vi "Least squares solution.vi"(0 "Y":T1 caption="Y（误差）", 5 "PWM数组":dbl[](array[numeric])) -> (2 "PWM8":dbl, 3 "PWM6":dbl, 4 "PWM1":dbl, 6 "PWM2":dbl, 8 "PWM3":dbl, 10 "PWM4":dbl, 13 "PWM9":dbl, 14 "PWM7":dbl, 15 "PWM5":dbl)   [LabVIEW 2017]
uses:
  <vilib>/Analysis/Matrix/Datatypes/RealMatrix.ctl
  <vilib>/Analysis/_algsub.llb/Real Matrix Condition Number.vi
  <vilib>/Analysis/baseanly.llb/Real A x B.vi
  <vilib>/Analysis/Matrix/Numeric/Add/Add - RM,RM.vi
  <vilib>/Analysis/baseanly.llb/Real Inverse Matrix.vi
  <vilib>/Analysis/NI_AALBase.lvlib
  <vilib>/Analysis/NI_AALPro.lvlib
  <vilib>/Analysis/Matrix/NI_Matrix.lvlib
panel:
  out "condition number 2":dbl caption="条件数" format="%.4f"
  out "x*y":dbl[][](array[numeric])
  out "A + B":T1
  out "condition number":dbl caption="条件数" format="%.4f"
  out "Inverse Matrix":T1 caption="逆矩阵"
  out "矩阵A x B":T1
  out "S表":dbl[][](array[numeric])
  out "X":T1 caption="X（pwm/灯塔pwm）"
  # "横坐标是灯板编号\n纵坐标是传感器编号"
  # "PWM的变化量"
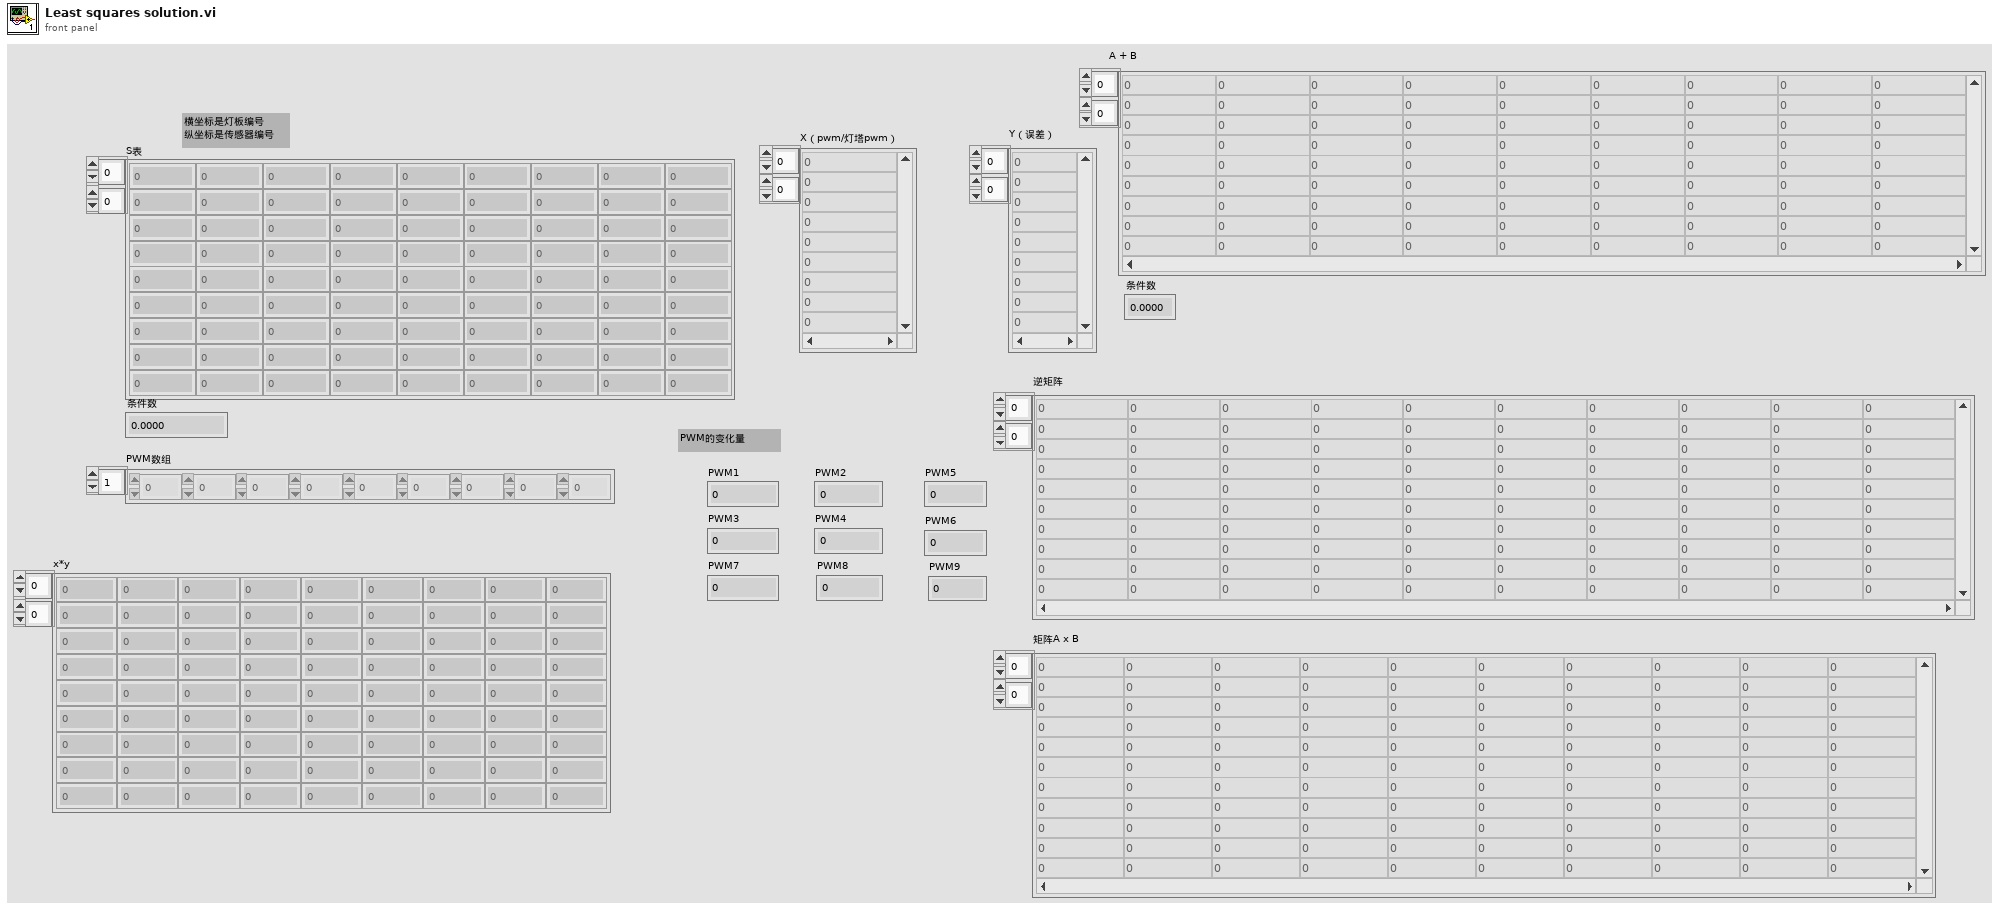
[diagram p1: front panel]
types:
  T1 = typedef "NI_Matrix.lvlib/RealMatrix.ctl" = dbl[][]
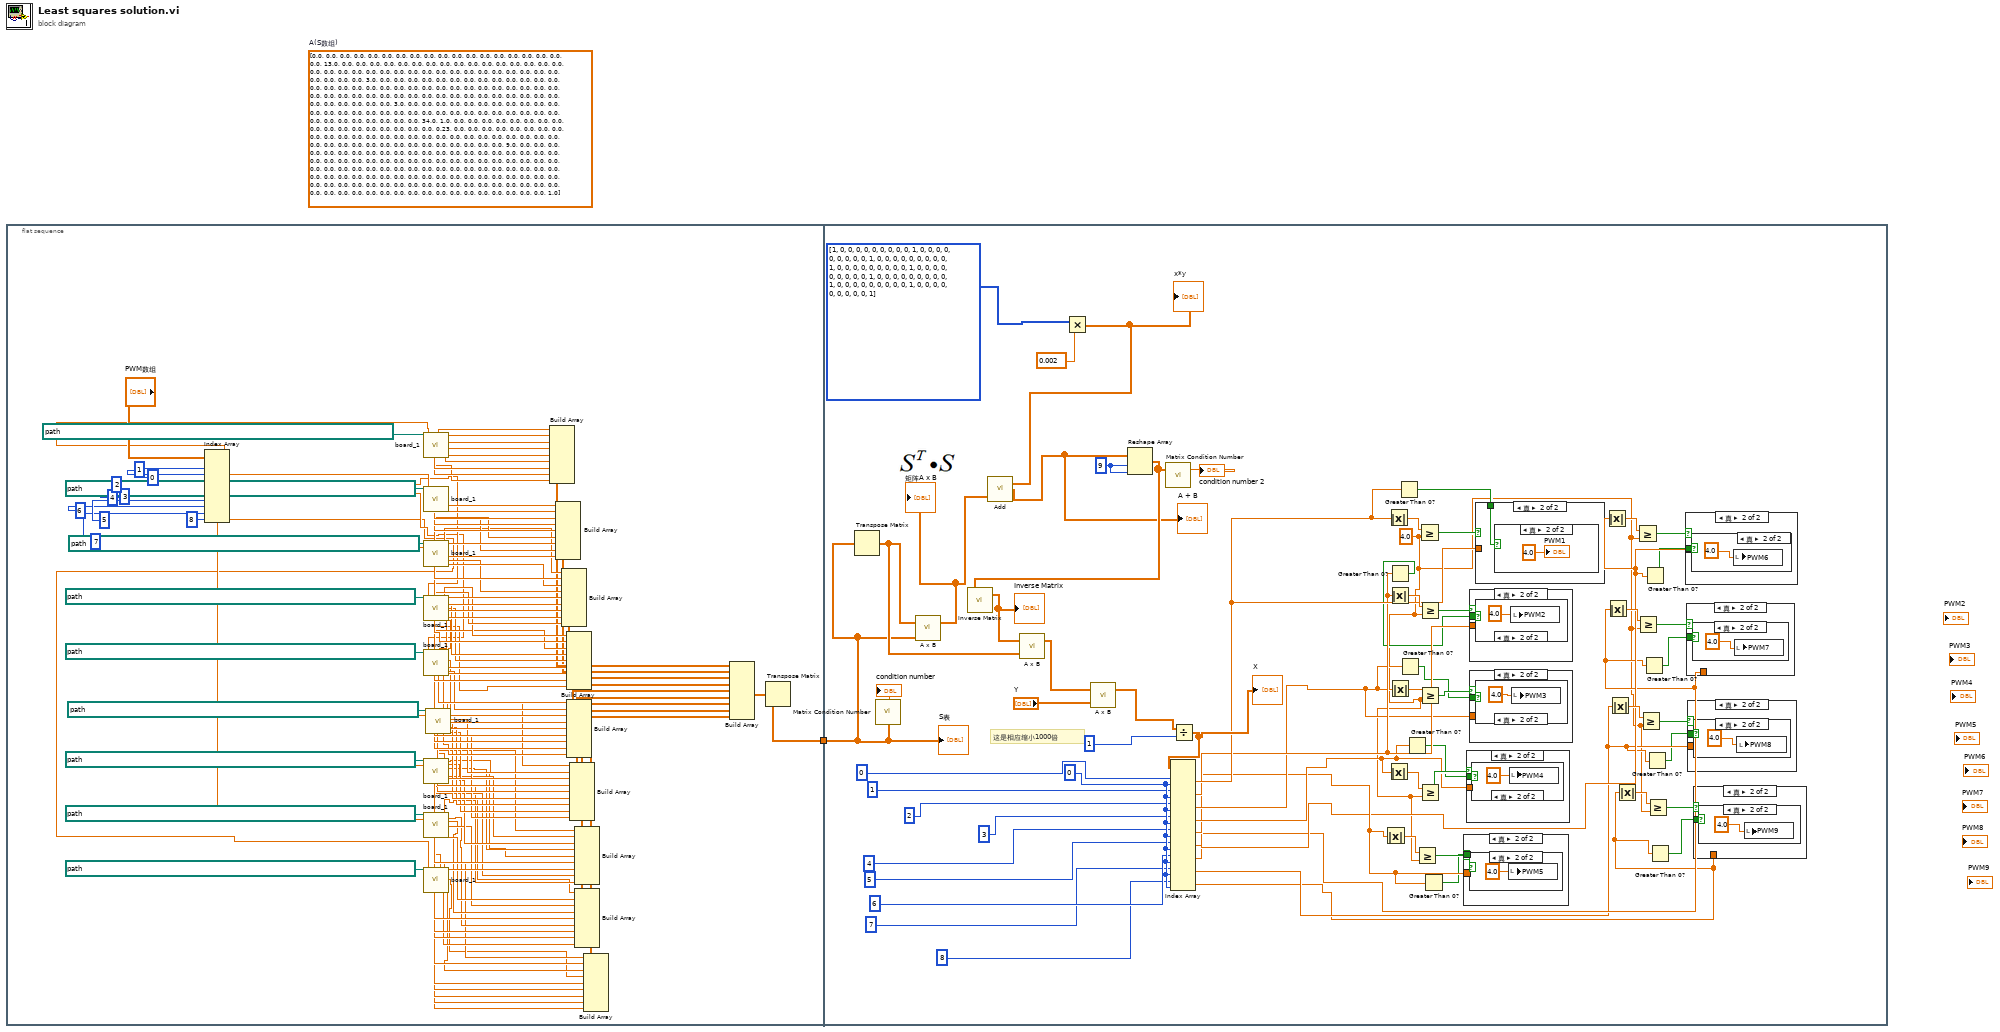
[diagram p0: block diagram]
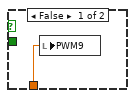
[diagram p2: hidden frame]
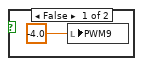
[diagram p3: hidden frame]
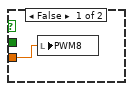
[diagram p4: hidden frame]
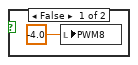
[diagram p5: hidden frame]
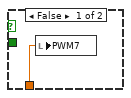
[diagram p6: hidden frame]
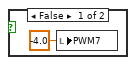
[diagram p7: hidden frame]
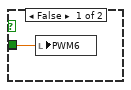
[diagram p8: hidden frame]
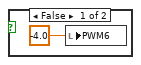
[diagram p9: hidden frame]
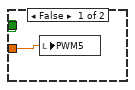
[diagram p10: hidden frame]
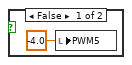
[diagram p11: hidden frame]
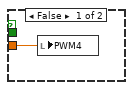
[diagram p12: hidden frame]
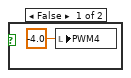
[diagram p13: hidden frame]
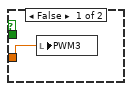
[diagram p14: hidden frame]
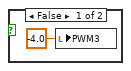
[diagram p15: hidden frame]
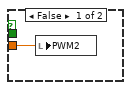
[diagram p16: hidden frame]
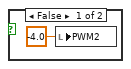
[diagram p17: hidden frame]
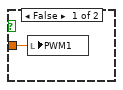
[diagram p18: hidden frame]
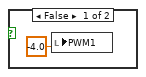
[diagram p19: hidden frame]
diagram:
  (unwired) dbl[][] [[0.0, 0.0, 0.0, 0.0, 0.0, 0.0, 0.0, 0.0, 0.0, 0.0, 0.0, 0.0, 0.0, 0.0, 0.0, 0.0, 0.0, 0.0], [0.0, 13.0, 0.0, 0.0, 0.0, 0.0, 0.0, 0.0, 0.0, 0.0, 0.0, 0.0, 0.0, 0.0, 0.0, 0.0, 0.0, 0.0], [0.0, 0.0, 0.0, 0.0, 0.0, 0.0, 0.0, 0.0, 0.0, 0.0, 0.0, 0.0, 0.0, 0.0, 0.0, 0.0, 0.0, 0.0], [0.0, 0.0, 0.0, 0.0, 3.0, 0.0, 0.0, 0.0, 0.0, 0.0, 0.0, 0.0, 0.0, 0.0, 0.0, 0.0, 0.0, 0.0], [0.0, 0.0, 0.0, 0.0, 0.0, 0.0, 0.0, 0.0, 0.0, 0.0, 0.0, 0.0, 0.0, 0.0, 0.0, 0.0, 0.0, 0.0], [0.0, 0.0, 0.0, 0.0, 0.0, 0.0, 0.0, 0.0, 0.0, 0.0, 0.0, 0.0, 0.0, 0.0, 0.0, 0.0, 0.0, 0.0], [0.0, 0.0, 0.0, 0.0, 0.0, 0.0, 3.0, 0.0, 0.0, 0.0, 0.0, 0.0, 0.0, 0.0, 0.0, 0.0, 0.0, 0.0], [0.0, 0.0, 0.0, 0.0, 0.0, 0.0, 0.0, 0.0, 0.0, 0.0, 0.0, 0.0, 0.0, 0.0, 0.0, 0.0, 0.0, 0.0], [0.0, 0.0, 0.0, 0.0, 0.0, 0.0, 0.0, 0.0, 34.0, 1.0, 0.0, 0.0, 0.0, 0.0, 0.0, 0.0, 0.0, 0.0], [0.0, 0.0, 0.0, 0.0, 0.0, 0.0, 0.0, 0.0, 0.0, 0.23, 0.0, 0.0, 0.0, 0.0, 0.0, 0.0, 0.0, 0.0], [0.0, 0.0, 0.0, 0.0, 0.0, 0.0, 0.0, 0.0, 0.0, 0.0, 0.0, 0.0, 0.0, 0.0, 0.0, 0.0, 0.0, 0.0], [0.0, 0.0, 0.0, 0.0, 0.0, 0.0, 0.0, 0.0, 0.0, 0.0, 0.0, 0.0, 0.0, 0.0, 9.0, 0.0, 0.0, 0.0], [0.0, 0.0, 0.0, 0.0, 0.0, 0.0, 0.0, 0.0, 0.0, 0.0, 0.0, 0.0, 0.0, 0.0, 0.0, 0.0, 0.0, 0.0], [0.0, 0.0, 0.0, 0.0, 0.0, 0.0, 0.0, 0.0, 0.0, 0.0, 0.0, 0.0, 0.0, 0.0, 0.0, 0.0, 0.0, 0.0], [0.0, 0.0, 0.0, 0.0, 0.0, 0.0, 0.0, 0.0, 0.0, 0.0, 0.0, 0.0, 0.0, 0.0, 0.0, 0.0, 0.0, 0.0], [0.0, 0.0, 0.0, 0.0, 0.0, 0.0, 0.0, 0.0, 0.0, 0.0, 0.0, 0.0, 0.0, 0.0, 0.0, 0.0, 0.0, 0.0], [0.0, 0.0, 0.0, 0.0, 0.0, 0.0, 0.0, 0.0, 0.0, 0.0, 0.0, 0.0, 0.0, 0.0, 0.0, 0.0, 0.0, 0.0], [0.0, 0.0, 0.0, 0.0, 0.0, 0.0, 0.0, 0.0, 0.0, 0.0, 0.0, 0.0, 0.0, 0.0, 0.0, 0.0, 0.0, 1.0]]  # A(S数组)
  n1 = flat-sequence {
    tunnel: [w11] -> w1
    tunnel: w1 -> [w125]
    frame #0 {
      n2 = Index Array(array="PWM数组", index #1=0 ("索引"), index #2=1 ("索引"), index #3=2 ("索引"), index #4=3 ("索引"), index #5=4 ("索引"), index #6=5 ("索引"), index #7=6 ("索引"), index #8=7 ("索引"), index #9=8 ("索引")) -> (element #1=w111:dbl, element #2=w19:dbl, element #3=w18:dbl, element #4=w17:dbl, element #5=w16:dbl, element #6=w15:dbl, element #7=w14:dbl, element #8=w13:dbl, element #9=w12:dbl)
      n3 = call "board_1.vi"("文件（使用对话框）"=path "D:/桌面文件/自动备份/自动匀光/程序/labview36/raw_data/S_rawdata_b1.txt", "PWM1"=w111) -> ("S1"=w110:dbl, "S2"=w109:dbl, "S3"=w108:dbl, "S4"=w107:dbl, "S5"=w106:dbl, "S6"=w105:dbl, "S7"=w104:dbl, "S8"=w103:dbl, "S9"=w102:dbl)  [unwired: 17 in]
      n4 = call "board_1.vi"("文件（使用对话框）"=path "D:/桌面文件/自动备份/自动匀光/程序/labview36/raw_data/S_rawdata_b2.txt", "PWM1"=w19) -> ("S1"=w101:dbl, "S2"=w100:dbl, "S3"=w99:dbl, "S4"=w98:dbl, "S5"=w97:dbl, "S6"=w96:dbl, "S7"=w95:dbl, "S8"=w94:dbl, "S9"=w93:dbl)  [unwired: 17 in]
      n5 = call "board_1.vi"("文件（使用对话框）"=path "D:/桌面文件/自动备份/自动匀光/程序/labview36/raw_data/S_rawdata_b3.txt", "PWM1"=w18) -> ("S1"=w92:dbl, "S2"=w91:dbl, "S3"=w90:dbl, "S4"=w89:dbl, "S5"=w88:dbl, "S6"=w87:dbl, "S7"=w86:dbl, "S8"=w85:dbl, "S9"=w84:dbl)  [unwired: 17 in]
      n6 = call "board_1.vi"("文件（使用对话框）"=path "D:/桌面文件/自动备份/自动匀光/程序/labview36/raw_data/S_rawdata_b4.txt", "PWM1"=w17) -> ("S1"=w83:dbl, "S2"=w82:dbl, "S3"=w81:dbl, "S4"=w80:dbl, "S5"=w79:dbl, "S6"=w78:dbl, "S7"=w77:dbl, "S8"=w76:dbl, "S9"=w75:dbl)  [unwired: 17 in]
      n7 = call "board_1.vi"("文件（使用对话框）"=path "D:/桌面文件/自动备份/自动匀光/程序/labview36/raw_data/S_rawdata_b5.txt", "PWM1"=w16) -> ("S1"=w74:dbl, "S2"=w73:dbl, "S3"=w72:dbl, "S4"=w71:dbl, "S5"=w70:dbl, "S6"=w69:dbl, "S7"=w68:dbl, "S8"=w67:dbl, "S9"=w66:dbl)  [unwired: 17 in]
      n8 = call "board_1.vi"("文件（使用对话框）"=path "D:/桌面文件/自动备份/自动匀光/程序/labview36/raw_data/S_rawdata_b7.txt", "PWM1"=w14) -> ("S1"=w56:dbl, "S2"=w55:dbl, "S3"=w54:dbl, "S4"=w53:dbl, "S5"=w52:dbl, "S6"=w51:dbl, "S7"=w50:dbl, "S8"=w49:dbl, "S9"=w48:dbl)  [unwired: 17 in]
      n9 = call "board_1.vi"("文件（使用对话框）"=path "D:/桌面文件/自动备份/自动匀光/程序/labview36/raw_data/S_rawdata_b8.txt", "PWM1"=w13) -> ("S1"=w47:dbl, "S2"=w46:dbl, "S3"=w45:dbl, "S4"=w44:dbl, "S5"=w43:dbl, "S6"=w42:dbl, "S7"=w41:dbl, "S8"=w40:dbl, "S9"=w39:dbl)  [unwired: 17 in]
      n10 = call "board_1.vi"("文件（使用对话框）"=path "D:/桌面文件/自动备份/自动匀光/程序/labview36/raw_data/S_rawdata_b9.txt", "PWM1"=w12) -> ("S1"=w30:dbl, "S2"=w29:dbl, "S3"=w28:dbl, "S4"=w27:dbl, "S5"=w26:dbl, "S6"=w25:dbl, "S7"=w24:dbl, "S8"=w23:dbl, "S9"=w22:dbl)  [unwired: 17 in]
      n11 = call "board_1.vi"("文件（使用对话框）"=path "D:/桌面文件/自动备份/自动匀光/程序/labview36/raw_data/S_rawdata_b6.txt", "PWM1"=w15) -> ("S1"=w65:dbl, "S2"=w64:dbl, "S3"=w63:dbl, "S4"=w62:dbl, "S5"=w61:dbl, "S6"=w60:dbl, "S7"=w59:dbl, "S8"=w58:dbl, "S9"=w57:dbl)  [unwired: 17 in]
      n12 = Build Array(w110, w109, w108, w107, w106, w105, w104, w103, w102) -> (w38:dbl[])
      n13 = Build Array(w101, w100, w99, w98, w97, w96, w95, w94, w93) -> (w37:dbl[])
      n14 = Build Array(w92, w91, w90, w89, w88, w87, w86, w85, w84) -> (w36:dbl[])
      n15 = Build Array(w83, w82, w81, w80, w79, w78, w77, w76, w75) -> (w35:dbl[])
      n16 = Build Array(w74, w73, w72, w71, w70, w69, w68, w67, w66) -> (w34:dbl[])
      n17 = Build Array(w65, w64, w63, w62, w61, w60, w59, w58, w57) -> (w33:dbl[])
      n18 = Build Array(w56, w55, w54, w53, w52, w51, w50, w49, w48) -> (w32:dbl[])
      n19 = Build Array(w47, w46, w45, w44, w43, w42, w41, w40, w39) -> (w31:dbl[])
      n20 = Build Array(w30, w29, w28, w27, w26, w25, w24, w23, w22) -> (w21:dbl[])
      n21 = Build Array(w38, w37, w36, w35, w34, w33, w32, w31, w21) -> (w20:dbl[][])
      n22 = Transpose Matrix(1:w20) -> (0:w11:dbl[][])
    }
    frame #1 {
      w131 = 9 ("维数大小")
      w122 = 4.0 ("y")
      w182 = 0 ("索引 (行)")
      # "这是相应缩小1000倍"
      n23 = Transpose Matrix(1:w125) -> (0:w184:dbl[][])
      n24 = call-poly <vilib>:"Matrix Condition Number.vi"("Input Matrix"=w125) -> ("condition number"=→"condition number":dbl)  [unwired: 1 in, 1 out]
      n25 = call-poly <vilib>:"A x B.vi"("B"=w125, "A"=w184) -> ("A x B"=w124:T1)  [unwired: 1 out]
      "矩阵A x B" <- w124
      n26 = Multiply(x=i32[][] [[1, 0, 0, 0, 0, 0, 0, 0, 0], [0, 1, 0, 0, 0, 0, 0, 0, 0], [0, 0, 1, 0, 0, 0, 0, 0, 0], [0, 0, 0, 1, 0, 0, 0, 0, 0], [0, 0, 0, 0, 1, 0, 0, 0, 0], [0, 0, 0, 0, 0, 1, 0, 0, 0], [0, 0, 0, 0, 0, 0, 1, 0, 0], [0, 0, 0, 0, 0, 0, 0, 1, 0], [0, 0, 0, 0, 0, 0, 0, 0, 1]], y=0.002) -> (x*y=w130:dbl[][])
      "x*y" <- w130
      n27 = call-poly <vilib>:"Add.vi"("Real Matrix B"=w124, "Real Matrix A"=w130) -> ("A + B"=w126:T1)
      "A + B" <- w126
      n28 = Reshape Array(w126, w131, w131) -> (w128:T1)
      n29 = call-poly <vilib>:"Inverse Matrix.vi"("Input Matrix"=w128) -> ("Inverse Matrix"=w183:T1)  [unwired: 1 in, 1 out]
      "Inverse Matrix" <- w183
      n30 = call-poly <vilib>:"A x B.vi"("B"=w184, "A"=w183) -> ("A x B"=w185:T1)  [unwired: 1 out]
      n31 = call-poly <vilib>:"A x B.vi"("B"="Y", "A"=w185) -> ("A x B"=w171:T1)  [unwired: 1 out]
      n32 = call-poly <vilib>:"Matrix Condition Number.vi"("Input Matrix"=w128) -> ("condition number"=→"condition number 2":dbl)  [unwired: 1 in, 1 out]
      n33 = Divide(x=w171, y=1) -> (x/y=w169:T1)
      "X" <- w169
      n34 = Index Array(array=w169, index (row) #1=0 ("禁用的索引 (列)"), index (col) #1=w182, index (row) #2=1 ("禁用的索引 (列)"), index (col) #2=w182, index (row) #3=2 ("禁用的索引 (列)"), index (col) #3=w182, index (row) #4=3 ("禁用的索引 (列)"), index (col) #4=w182, index (row) #5=4 ("禁用的索引 (列)"), index (col) #5=w182, index (row) #6=5 ("禁用的索引 (列)"), index (col) #6=w182, index (row) #7=6 ("禁用的索引 (列)"), index (col) #7=w182, index (row) #8=7 ("禁用的索引 (列)"), index (col) #8=w182, index (row) #9=8 ("禁用的索引 (列)"), index (col) #9=w182) -> (element #1=w150:dbl, element #2=w148:dbl, element #3=w146:dbl, element #4=w144:dbl, element #5=w142:dbl, element #6=w140:dbl, element #7=w138:dbl, element #8=w136:dbl, element #9=w134:dbl)
      n35 = Absolute Value(x=w142) -> (abs(x)=w161:dbl)
      n36 = Absolute Value(x=w150) -> (abs(x)=w168:dbl)
      n37 = Absolute Value(x=w144) -> (abs(x)=w162:dbl)
      n38 = Absolute Value(x=w148) -> (abs(x)=w165:dbl)
      n39 = Greater Than 0?(x=w148) -> (x > 0?=w147:bool)
      n40 = Absolute Value(x=w146) -> (abs(x)=w164:dbl)
      n41 = Greater Than 0?(x=w150) -> (x > 0?=w149:bool)
      n42 = Greater Than 0?(x=w146) -> (x > 0?=w145:bool)
      n43 = Greater Than 0?(x=w144) -> (x > 0?=w143:bool)
      n44 = Greater Or Equal?(x=w161, y=w122) -> (x >= y?=w160:bool)
      n45 = Greater Or Equal?(x=w168, y=w122) -> (x >= y?=w167:bool)
      n46 = Greater Or Equal?(x=w165, y=w122) -> (x >= y?=w166:bool)
      n47 = Greater Or Equal?(x=w164, y=w122) -> (x >= y?=w163:bool)
      n48 = Greater Or Equal?(x=w162, y=w122) -> (x >= y?=w151:bool)
      n49 = Greater Than 0?(x=w142) -> (x > 0?=w141:bool)
      n50 = case shown="真" w160 {
        tunnel: w142 -> [w202 _]
        tunnel: w141 -> [_ w203]
        frame False {
          n51 = local write "PWM5"(w202) -> ()
        }
        frame True {
          n52 = case shown="真" w203 {
            frame False {
              n53 = local write "PWM5"(-4.0 ("PWM5")) -> ()
            }
            frame True {
              n54 = local write "PWM5"(4.0 ("PWM1")) -> ()
            }
          }
        }
      }
      n55 = case shown="真" w151 {
        tunnel: w144 -> [w206 _]
        tunnel: w143 -> [_ w207]
        frame False {
          n56 = local write "PWM4"(w206) -> ()
        }
        frame True {
          n57 = case shown="真" w207 {
            frame False {
              n58 = local write "PWM4"(-4.0 ("PWM4")) -> ()
            }
            frame True {
              n59 = local write "PWM4"(4.0 ("PWM1")) -> ()
            }
          }
        }
      }
      n60 = case shown="真" w166 {
        tunnel: w148 -> [w214 _]
        tunnel: w147 -> [_ w215]
        frame False {
          n61 = local write "PWM2"(w214) -> ()
        }
        frame True {
          n62 = case shown="真" w215 {
            frame False {
              n63 = local write "PWM2"(-4.0 ("PWM2")) -> ()
            }
            frame True {
              n64 = local write "PWM2"(4.0 ("PWM1")) -> ()
            }
          }
        }
      }
      n65 = case shown="真" w163 {
        tunnel: w146 -> [w210 _]
        tunnel: w145 -> [_ w211]
        frame False {
          n66 = local write "PWM3"(w210) -> ()
        }
        frame True {
          n67 = case shown="真" w211 {
            frame False {
              n68 = local write "PWM3"(-4.0 ("PWM3")) -> ()
            }
            frame True {
              n69 = local write "PWM3"(4.0 ("PWM1")) -> ()
            }
          }
        }
      }
      n70 = case shown="真" w167 {
        tunnel: w150 -> [w218 _]
        tunnel: w149 -> [_ w219]
        frame False {
          n71 = local write "PWM1"(w218) -> ()
        }
        frame True {
          n72 = case shown="真" w219 {
            frame False {
              n73 = local write "PWM1"(-4.0 ("PWM1")) -> ()
            }
            frame True {
              "PWM1" <- 4.0 ("PWM1")
            }
          }
        }
      }
      n74 = Absolute Value(x=w140) -> (abs(x)=w158:dbl)
      n75 = Absolute Value(x=w138) -> (abs(x)=w157:dbl)
      n76 = Absolute Value(x=w136) -> (abs(x)=w154:dbl)
      n77 = Absolute Value(x=w134) -> (abs(x)=w153:dbl)
      n78 = Greater Or Equal?(x=w158, y=w122) -> (x >= y?=w159:bool)
      n79 = Greater Or Equal?(x=w157, y=w122) -> (x >= y?=w156:bool)
      n80 = Greater Or Equal?(x=w154, y=w122) -> (x >= y?=w155:bool)
      n81 = Greater Than 0?(x=w138) -> (x > 0?=w137:bool)
      n82 = Greater Than 0?(x=w140) -> (x > 0?=w139:bool)
      n83 = Greater Than 0?(x=w136) -> (x > 0?=w135:bool)
      n84 = Greater Or Equal?(x=w153, y=w122) -> (x >= y?=w152:bool)
      n85 = Greater Than 0?(x=w134) -> (x > 0?=w133:bool)
      n86 = case shown="真" w159 {
        tunnel: w140 -> [w198 _]
        tunnel: w139 -> [_ w199]
        frame False {
          n87 = local write "PWM6"(w198) -> ()
        }
        frame True {
          n88 = case shown="真" w199 {
            frame False {
              n89 = local write "PWM6"(-4.0 ("PWM5")) -> ()
            }
            frame True {
              n90 = local write "PWM6"(4.0 ("PWM1")) -> ()
            }
          }
        }
      }
      n91 = case shown="真" w156 {
        tunnel: w138 -> [w194 _]
        tunnel: w137 -> [_ w195]
        frame False {
          n92 = local write "PWM7"(w194) -> ()
        }
        frame True {
          n93 = case shown="真" w195 {
            frame False {
              n94 = local write "PWM7"(-4.0 ("PWM5")) -> ()
            }
            frame True {
              n95 = local write "PWM7"(4.0 ("PWM1")) -> ()
            }
          }
        }
      }
      n96 = case shown="真" w155 {
        tunnel: w136 -> [w190 _]
        tunnel: w135 -> [_ w191]
        frame False {
          n97 = local write "PWM8"(w190) -> ()
        }
        frame True {
          n98 = case shown="真" w191 {
            frame False {
              n99 = local write "PWM8"(-4.0 ("PWM5")) -> ()
            }
            frame True {
              n100 = local write "PWM8"(4.0 ("PWM1")) -> ()
            }
          }
        }
      }
      n101 = case shown="真" w152 {
        tunnel: w134 -> [w186 _]
        tunnel: w133 -> [_ w187]
        frame False {
          n102 = local write "PWM9"(w186) -> ()
        }
        frame True {
          n103 = case shown="真" w187 {
            frame False {
              n104 = local write "PWM9"(-4.0 ("PWM5")) -> ()
            }
            frame True {
              n105 = local write "PWM9"(4.0 ("PWM1")) -> ()
            }
          }
        }
      }
      "S表" <- w125
    }
  }
